vi "Detect_Application_Kind.vi"(8 "error in":errorcluster) -> (0 "error out":errorcluster, 1 "Application:Kind":T1(ring), 3 "Development System":bool)   [LabVIEW 2020]
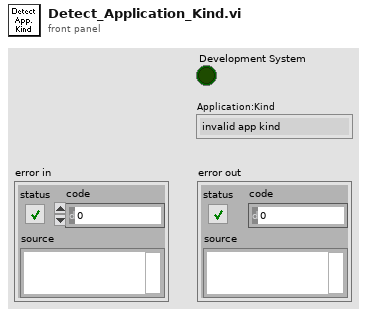
[diagram p1: front panel]
types:
  T1 = enum32{"invalid app kind", "Development System", "Run Time System", "Student Edition", "Embedded LabVIEW", "Evaluation", "Custom"}
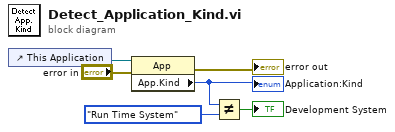
[diagram p0: block diagram]
diagram:
  n1 = control-ref of="This Application"() -> (w2:refnum<vi>)
  n2 = property class="App"(reference=w2, error in="error in") -> (error out=→"error out":errorcluster, "App.Kind"=w4:T1)  [unwired: 1 out]
  "Application:Kind" <- w4
  n3 = Not Equal?(x=w4, y=T1."Run Time System" ("Application:Kind")) -> (x != y?=→"Development System":bool)
